vi "myRIO_BRig_RT_TCP__v2.vi"(0 "input_hTCP":refnum<k5>, 1 "input_AI1":i16, 2 "input_AI0":i16, 3 "input_I_connected_TCP":bool, 5 "input_iBlock":u16, 7 "input_spout":enum16{"Left", "Right"}(ring), 9 "input_iTrial":u16, 11 "input_error":errorcluster, 13 "input_iState":T1) -> (4 "output_hTCP":refnum<k5>, 15 "output_error":errorcluster)   [LabVIEW 2014]
uses:
  myRIO_BRig_RT__Case_Exp_stateList.ctl
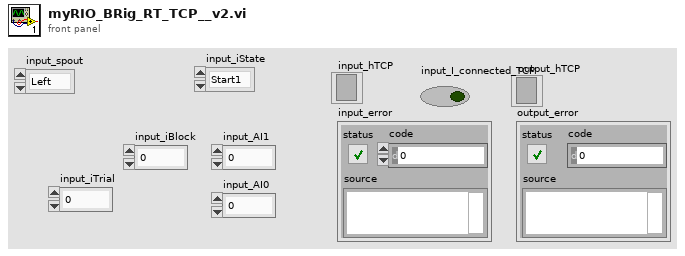
[diagram p1: front panel]
types:
  T1 = typedef "myRIO_BRig_RT__Case_Exp_stateList.ctl" = enum16{"Start1", "Start2", "Start3", "saveSettings1", "saveSettings2", "saveSettings3", "saveSettings4_LC_ENL", "saveSettings5_LC_Cue", "saveSettings6_LC_Other", "setSettings_Audio", "setSettings_Laser", "initBlock_pre", "initBlock", "initBlock2", "initBlock_post", "initTrial_pre", "initTrial", "initTrial2", "initTrial3", "initTrial4", "initTrial_LC_ENL1", "initTrial_LC_Cue1", "initTrial_LC_Sel", "initTrial_post", "ENL1_pre", "ENL1", "ENL1_post", "ENL1Penalty_pre", "ENL1Penalty", "ENL2_pre", "ENL2", "ENL2Penalty_pre", "ENL2Penalty", "Cue1_pre", "Cue1", "Cue1_post", "Cue1Penalty_pre", "Cue1Penalty", "Cue2_pre", "Cue2", "Cue2Penalty_pre", "Cue2Penalty", "Selection_pre", "Selection", "Select_post", "SelectReward_pre", "SelectReward", "SelectRewardPost_pre", "SelectRewardPost", "SelectWrong_pre", "SelectWrong", "SelectWrong_post", "SelectTimeout_pre", "SelectTimeout", "SelectTimeout_post", "endTrial_pre", "endTrial1", "endTrial2", "endTrial3", "endTrial_post", "endBlock_pre", "endBlock", "endBlock_post", "endExp", "commConnect", "commUpload_pre", "commUpload_dataBlock", "commUpload_dataCurrent", "commUpload_dataExp", "commUpload_dataLC", "commUpload_dataTrial", "commUpload_post", "saveData_pre", "saveData_dataBlock", "saveData_dataCurrent", "saveData_dataExp", "saveData_dataLC", "saveData_dataTrial", "saveData_post", "empty_endBlock1", "empty_endBlock2", "empty_endTrial1", "empty_endTrial2", "empty_endTrial3", "empty_endTrial4", "empty_endTrial5", "dummyState", "dummyState_endBlock"}
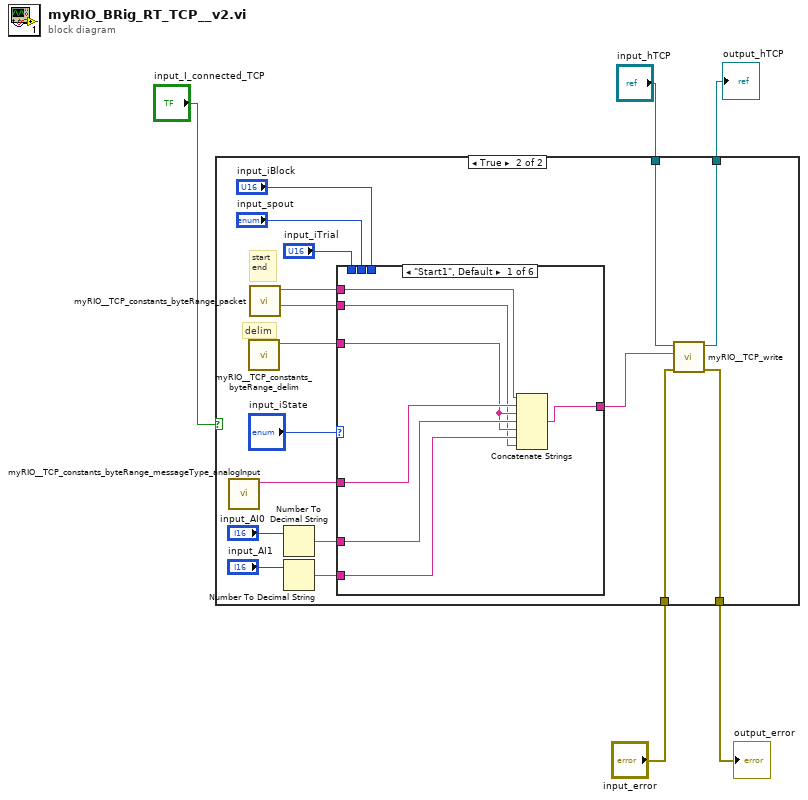
[diagram p0: block diagram]
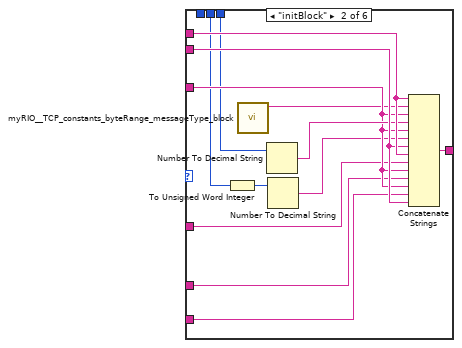
[diagram p3: hidden frame]
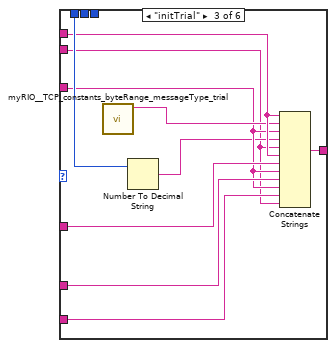
[diagram p4: hidden frame]
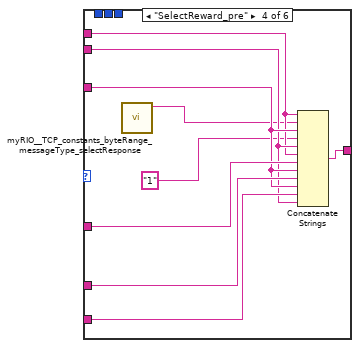
[diagram p5: hidden frame]
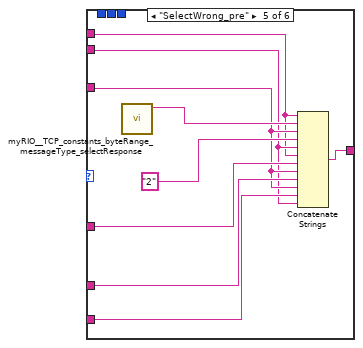
[diagram p6: hidden frame]
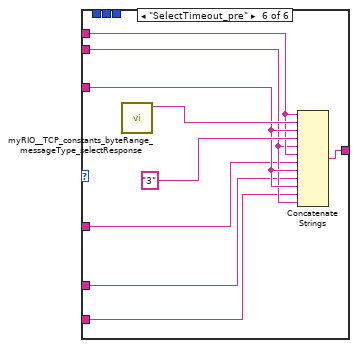
[diagram p7: hidden frame]
diagram:
  n1 = case shown="True" "input_I_connected_TCP" {
    tunnel: "input_hTCP" -> [w7 w24]
    tunnel: "input_error" -> [w6 w23]
    tunnel: [w7 w22] -> w3
    tunnel: [w6 w21] -> w2
    frame False {
    }
    frame True {
      # "start\nend"
      # "delim"
      n2 = call "myRIO__TCP_constants_byteRange_messageType_analogInput.vi"() -> ("output_analogInput_char"=w11:string)  [unwired: 10 in, 1 out]
      n3 = call "myRIO__TCP_constants_byteRange_delim.vi"() -> ("output_delim_char"=w17:string)  [unwired: 10 in, 1 out]
      n4 = call "myRIO__TCP_constants_byteRange_packet.vi"() -> ("output_end_char"=w18:string, "output_start_char"=w19:string)  [unwired: 8 in, 2 out]
      n5 = Number To Decimal String(number="input_AI0") -> (decimal integer string=w13:string)  [unwired: 1 in]
      n6 = Number To Decimal String(number="input_AI1") -> (decimal integer string=w12:string)  [unwired: 1 in]
      n7 = case shown="\"Start1\", Default" "input_iState" {
        tunnel: w19 -> [w31 w42 w49 w57 w64 w77]
        tunnel: w18 -> [w26 w41 w45 w58 w65 w76]
        tunnel: w17 -> [w28 w39 w47 w59 w66 w78]
        tunnel: [w25 w43 w54 w60 w70 w79] -> w16
        tunnel: w13 -> [w29 w37 w52 w62 w68 w74]
        tunnel: w12 -> [w27 w36 w51 w61 w69 w73]
        tunnel: w11 -> [w30 w35 w53 w63 w67 w75]
        tunnel: "input_iTrial" -> [_ _ w50 _ _ _]
        tunnel: "input_spout" -> [_ w33 _ _ _ _]
        tunnel: "input_iBlock" -> [_ w34 _ _ _ _]
        frame "Start1", Default {
          n8 = Concatenate Strings(w31, w30, w28, w29, w28, w27, w26) -> (w25:string)
        }
        frame "initBlock" {
          n9 = To Unsigned Word Integer(number=w33) -> (unsigned 16bit integer=w44:u16)
          n10 = call "myRIO__TCP_constants_byteRange_messageType_block.vi"() -> ("output_Block_char"=w32:string)  [unwired: 10 in, 1 out]
          n11 = Number To Decimal String(number=w34) -> (decimal integer string=w40:string)  [unwired: 1 in]
          n12 = Number To Decimal String(number=w44) -> (decimal integer string=w38:string)  [unwired: 1 in]
          n13 = Concatenate Strings(w42, w32, w39, w40, w39, w38, w41, w42, w35, w39, w37, w39, w36, w41) -> (w43:string)
        }
        frame "initTrial" {
          n14 = call "myRIO__TCP_constants_byteRange_messageType_trial.vi"() -> ("output_Trial_char"=w48:string)  [unwired: 10 in, 1 out]
          n15 = Number To Decimal String(number=w50) -> (decimal integer string=w46:string)  [unwired: 1 in]
          n16 = Concatenate Strings(w49, w48, w47, w46, w45, w49, w53, w47, w52, w47, w51, w45) -> (w54:string)
        }
        frame "SelectReward_pre" {
          n17 = call "myRIO__TCP_constants_byteRange_messageType_selectResponse.vi"() -> ("output_selectResponse_char"=w55:string)  [unwired: 10 in, 1 out]
          n18 = Concatenate Strings(w57, w55, w59, "1", w58, w57, w63, w59, w62, w59, w61, w58) -> (w60:string)
        }
        frame "SelectWrong_pre" {
          n19 = call "myRIO__TCP_constants_byteRange_messageType_selectResponse.vi"() -> ("output_selectResponse_char"=w71:string)  [unwired: 10 in, 1 out]
          n20 = Concatenate Strings(w64, w71, w66, "2", w65, w64, w67, w66, w68, w66, w69, w65) -> (w70:string)
        }
        frame "SelectTimeout_pre" {
          n21 = call "myRIO__TCP_constants_byteRange_messageType_selectResponse.vi"() -> ("output_selectResponse_char"=w80:string)  [unwired: 10 in, 1 out]
          n22 = Concatenate Strings(w77, w80, w78, "3", w76, w77, w75, w78, w74, w78, w73, w76) -> (w79:string)
        }
      }
      n23 = call "myRIO__TCP_write.vi"("input_error"=w23, "input_packet"=w16, "input_hTCP"=w24) -> ("output_error"=w21:errorcluster, "output_hTCP"=w22:refnum<k5>)  [unwired: 6 in, 1 out]
    }
  }
  "output_hTCP" <- w3
  "output_error" <- w2
